vi "Obtain C-Scan Build Up Value.vi"(8 "A-Scans":dbl[](array[numeric]), 11 "C-Scan Build Up Quantity":T1(radio)) -> (2 "Desired Value for C-Scan":dbl)   [LabVIEW 2020]
doc: "Performs the required data procecssing on the A-scans to obtain the desired value to build up the C-scan image\n\nArgs:\n\nC-Scan Build Up Quality - User's input on which quantity to build up image on\nA-Scans - Incoming A-scans to be processed\n\nReturns:\nDesired Value for C-Scan - Individual data point with the key characteristic for that scanning point. Used to create entire C-scan"
uses:
  <vilib>/Analysis/2dsp.llb/Integral Method.ctl
  <vilib>/Analysis/8numeric.llb/1D Numeric Integration.vi
  <vilib>/Analysis/NI_AALPro.lvlib
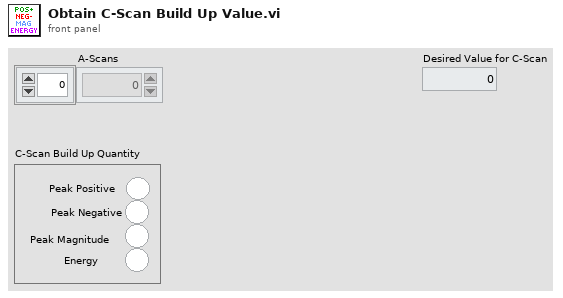
[diagram p1: front panel]
types:
  T1 = enum32{"No Selection", "Peak Positive", "Peak Negative", "Peak Magnitude", "Energy"}
  T2 = typedef "NI_AALPro.lvlib/Integral Method.ctl" = i32
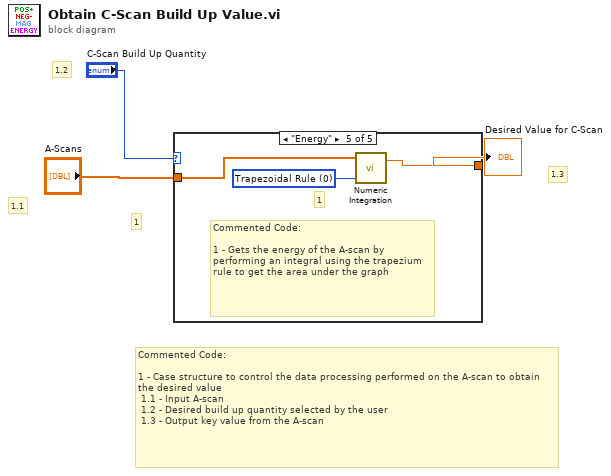
[diagram p0: block diagram]
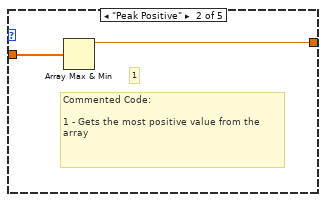
[diagram p3: hidden frame]
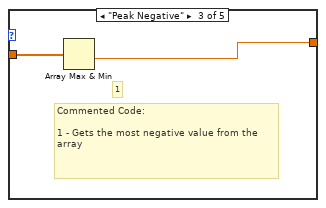
[diagram p4: hidden frame]
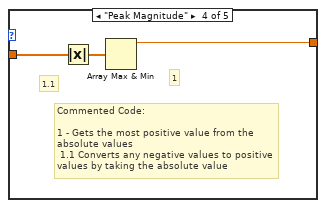
[diagram p5: hidden frame]
diagram:
  # "1"
  # "1.3"
  # "1.2"
  # "1.1"
  # "Commented Code:\n\n1 - Case structure to control the data processing performed on the A-scan to obtain the desired value\n 1.1 - Input A-scan\n 1.2 - Desired build up quantity selected by the user\n 1.3 - Output key value from the A-scan"
  n1 = case shown="\"Energy\"" "C-Scan Build Up Quantity" {
    tunnel: "A-Scans" -> [_ w5 w7 w10 w13]
    tunnel: [_ w4 w6 w8 w12] -> w2
    frame "No Selection" {
    }
    frame "Peak Positive" {
      # "1"
      # "Commented Code:\n\n1 - Gets the most positive value from the array"
      n2 = Array Max & Min(array=w5) -> (max value=w4:dbl)  [unwired: 3 out]
    }
    frame "Peak Negative" {
      # "Commented Code:\n\n1 - Gets the most negative value from the array"
      # "1"
      n3 = Array Max & Min(array=w7) -> (min value=w6:dbl)  [unwired: 3 out]
    }
    frame "Peak Magnitude" {
      # "Commented Code:\n\n1 - Gets the most positive value from the absolute values\n 1.1 Converts any negative values to positive values by taking the absolute value"
      # "1.1"
      # "1"
      n4 = Absolute Value(x=w10) -> (abs(x)=w9:dbl[])
      n5 = Array Max & Min(array=w9) -> (max value=w8:dbl)  [unwired: 3 out]
    }
    frame "Energy" {
      w11 = T2 0 items=["Trapezoidal Rule", "Simpson's Rule", "Simpson's 3/8 Rule", "Bode Rule"] ("integration method")
      # "Commented Code:\n\n1 - Gets the energy of the A-scan by performing an integral using the trapezium rule to get the area under the graph"
      # "1"
      n6 = call-poly <vilib>:"Numeric Integration.vi"("integration method"=w11, "Input Array"=w13) -> ("result"=w12:dbl)  [unwired: 1 in, 1 out]
    }
  }
  "Desired Value for C-Scan" <- w2
